vi "Ctor.vi"(8 "error in (no error)":errorcluster) -> (0 "error out":errorcluster, 3 "Results out":refnum<class "Results.lvclass">)   [LabVIEW 2020, in "Tester.lvlib" / "Results.lvclass"]
uses:
  Results.lvclass
  Results Ref.ctl
  Entry.ctl
  Result.ctl
  Results.lvclass/Results.ctl
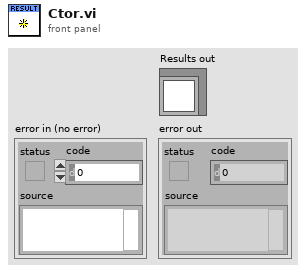
[diagram p1: front panel]
types:
  T1 = typedef "Tester.lvlib/Results.lvclass/Results Ref.ctl" = cluster{"Entries":T2[], "Overall Result":T3}
  T2 = typedef "Tester.lvlib/Results.lvclass/Entry.ctl" = cluster{"Name":string, "Value":variant, "Result":T3}
  T3 = typedef "Tester.lvlib/Results.lvclass/Result.ctl" = enum16{"No Result", "Pass", "Fail", "Error", "Abort"}
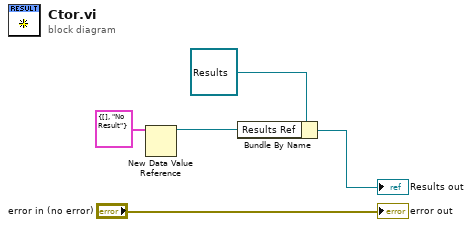
[diagram p0: block diagram]
diagram:
  n1 = New Data Value Reference(data value=T1 {"Entries"=[], "Overall Result"=enum."No Result"} ("Results Ref")) -> (data value reference=w1:refnum<data-value>)  [unwired: 1 in, 1 out]
  n2 = Bundle By Name(cluster=refnum<class "Results.lvclass"> refnum ("Results in"), "Results Ref"=w1) -> (→"Results out":refnum<class "Results.lvclass">)
  "error out" <- "error in (no error)"
